vi "read config.vi"(8 "error in (no error)":errorcluster, 10 "Config File Path":path, 11 "Stepper in":refnum<class "Stepper.lvclass">) -> (0 "error out":errorcluster, 3 "Stepper out":refnum<class "Stepper.lvclass">)   [LabVIEW 2025, in "Motor.lvlib" / "Stepper.lvclass"]
uses:
  Stepper.lvclass
  Stepper.lvclass/Stepper.ctl
  42028d02-6164-49c2-8705-dd9fbd1502b7.vi
  <vilib>/JDP Science/JSONtext/JSON text to Variant.vi
  <vilib>/JDP Science/JSONtext/LVClass Serializer/JSONtext LVClass Serializer.lvclass
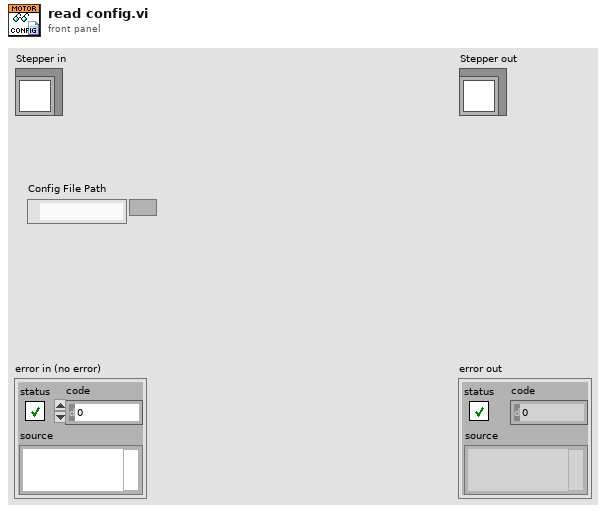
[diagram p1: front panel]
types:
  T1 = cluster{"Modbus_Param":cluster{"COM_Port":string, "Baud_Rate":i32, "Unit_ID":i32, "parity":i32, "flow_control":i32}}
  T2 = cluster{"COM_Port":string, "Baud_Rate":i32, "Unit_ID":i32, "parity":i32, "flow_control":i32}
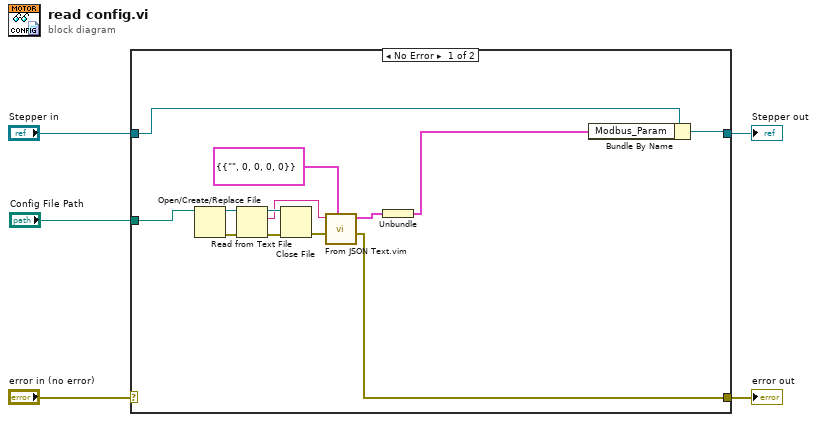
[diagram p0: block diagram]
diagram:
  n1 = case shown="No Error" "error in (no error)" {
    selector: "error in (no error)" -> [_ w20]
    tunnel: [w9 w20] -> w4
    tunnel: [w18 w19] -> w2
    tunnel: "Stepper in" -> [w17 w19]
    tunnel: "Config File Path" -> [w14 _]
    frame No Error {
      n2 = Open/Create/Replace File(file path (use dialog)=w14) -> (refnum out=w13:refnum<file>, error out=w16:errorcluster)  [unwired: 5 in, 1 out]
      n3 = Read from Text File(file (use dialog)=w13, error in=w16) -> (refnum out=w12:refnum<file>, text=w11:string, error out=w15:errorcluster)  [unwired: 2 in, 1 out]
      n4 = Close File(refnum=w12, error in=w15) -> (error out=w10:errorcluster)  [unwired: 1 out]
      n5 = call "From JSON Text.vim"("Data Type and Default Value"=T1 {"Modbus_Param"={"COM_Port"="", "Baud_Rate"=0, "Unit_ID"=0, "parity"=0, "flow_control"=0}}, "error in (no error)"=w10, "JSON"=w11) -> ("error out"=w9:errorcluster, "Data out"=w7:T1)  [unwired: 7 in]
      n6 = Unbundle(w7) -> ("Modbus_Param"=w6:T2)
      n7 = Bundle By Name(cluster=w17, "Modbus_Param"=w6) -> (w18:refnum<class "Stepper.lvclass">)
    }
    frame Error {
    }
  }
  "error out" <- w4
  "Stepper out" <- w2
